vi "Insert Data sub_ UT.vi"(8 "error in (no error)":errorcluster, 10 "y":i32, 11 "TableLogger_SQLite_Actor in":refnum<class "TableLogger_SQLite_Actor.lvclass">) -> (0 "error out":errorcluster, 2 "Insert?T":bool, 3 "TableLogger_SQLite_Actor out":refnum<class "TableLogger_SQLite_Actor.lvclass">)   [LabVIEW 2014, in "TableLogger_SQLite_Actor.lvlib" / "TableLogger_SQLite_Actor.lvclass"]
uses:
  TableLogger_SQLite_Actor.lvclass
  TableLogger_SQLite_Actor.lvclass/TableLogger_SQLite_Actor.ctl
  <vilib>/drjdpowell/SQLite Library/SQL Connection/Execute SQL (Single Integer).vi
  <vilib>/drjdpowell/SQLite Library/SQLite.lvlib
  <vilib>/drjdpowell/SQLite Library/SQL Connection/Connection.lvclass
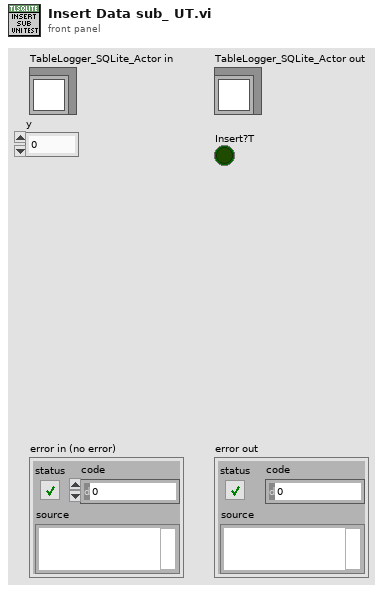
[diagram p1: front panel]
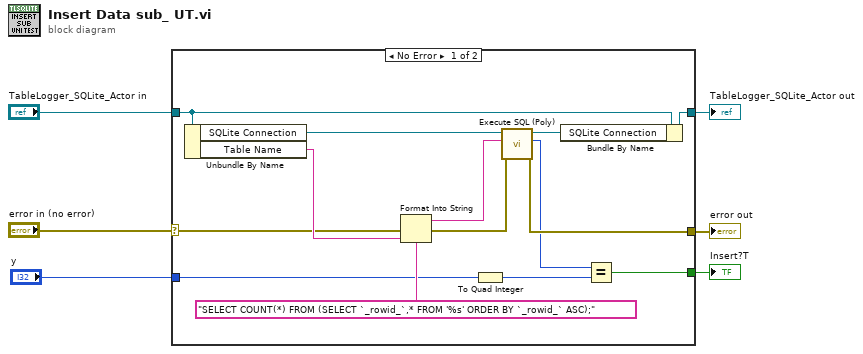
[diagram p0: block diagram]
diagram:
  n1 = case shown="No Error" "error in (no error)" {
    selector: "error in (no error)" -> [w10 w22]
    tunnel: [w20 w21] -> w6
    tunnel: "TableLogger_SQLite_Actor in" -> [w19 w21]
    tunnel: [w16 _] -> w3
    tunnel: [w14 w22] -> w2
    tunnel: "y" -> [w8 _]
    frame No Error {
      n2 = Unbundle By Name(w19) -> ("SQLite Connection"=w13:refnum<class "Connection.lvclass">, "Table Name"=w15:string)
      n3 = Format Into String(format string="SELECT COUNT(*) FROM (SELECT `_rowid_`,* FROM '%s' ORDER BY `_rowid_` ASC);" ("SQL"), error in=w10, w15) -> (resulting string=w11:string, error out=w17:errorcluster)  [unwired: 1 in]
      n4 = To Quad Integer(1:w8) -> (0:w7:i64)
      n5 = call-poly <vilib>:"Execute SQL (Poly).vi"("error in (no error)"=w17, "SQL"=w11, "SQLite Connection in"=w13) -> ("error out"=w14:errorcluster, "Result"=w9:i64, "SQLite Connection"=w18:refnum<class "Connection.lvclass">)  [unwired: 6 in]
      n6 = Bundle By Name(cluster=w19, "SQLite Connection"=w18) -> (w20:refnum<class "TableLogger_SQLite_Actor.lvclass">)
      n7 = Equal?(x=w9, y=w7) -> (x = y?=w16:bool)
    }
    frame Error {
    }
  }
  "Insert?T" <- w3
  "TableLogger_SQLite_Actor out" <- w6
  "error out" <- w2
